vi "Test Harvard pump control.vi"() -> ()   [LabVIEW 2014]
uses:
  <vilib>/Instr/_visa.llb/VISA Configure Serial Port (Instr).vi
panel:
  out "length":i32
  out "error out":errorcluster
  out "read buffer":string
  in  "Send string":string
  in  "stop":bool
  in  "Send string":bool
  out "command string sent":string
  in  "VISA resource name":refnum<visa-resource-name>="COM4"
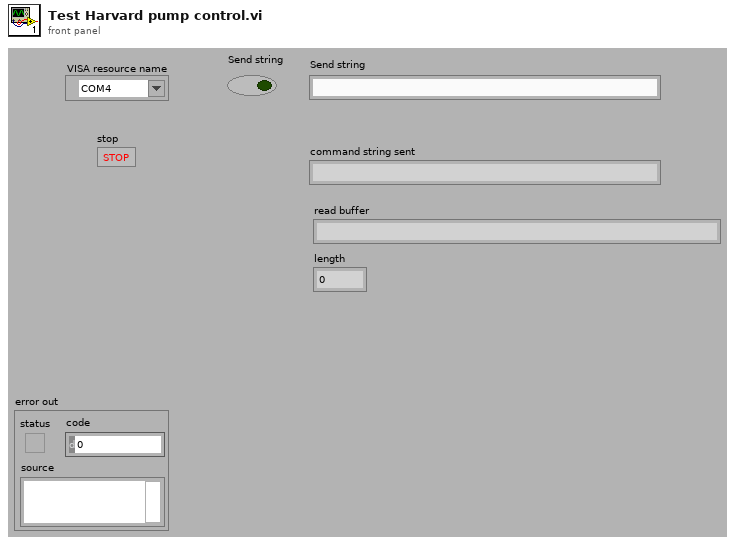
[diagram p1: front panel]
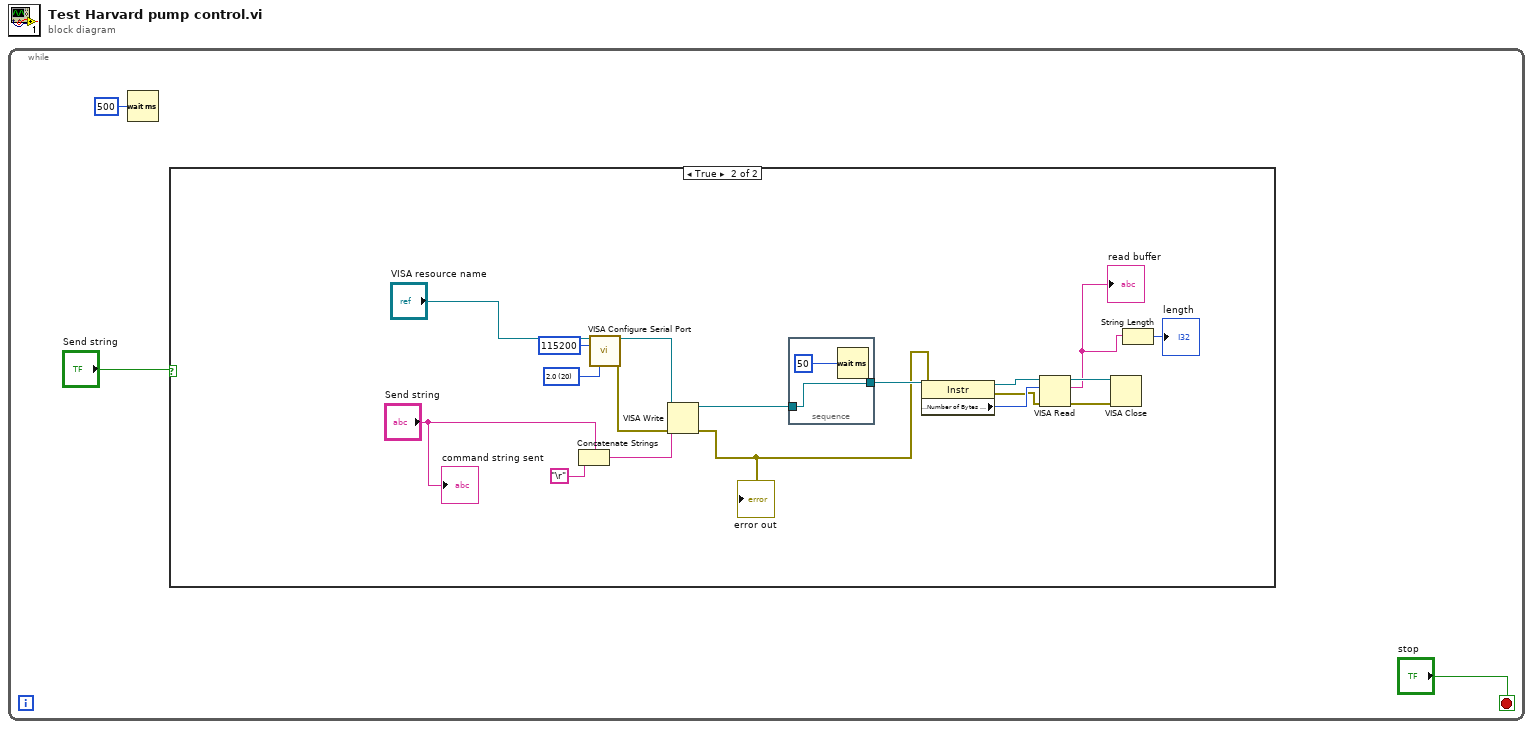
[diagram p0: block diagram]
diagram:
  n1 = while {
    stop <- "stop" stop-if-true
    n2 = Wait (ms)(milliseconds to wait=u32 500) -> ()  [unwired: 1 out]
    n3 = case shown="True" "Send string" {
      frame False {
      }
      frame True {
        w6 = u16 20 items=["1.0"=10, "1.5"=15, "2.0"=20] ("stop bits (10: 1 bit)")
        n4 = Concatenate Strings("Send string", "\r") -> (w16:string)
        n5 = call-poly "VISA Configure Serial Port"("VISA resource name"="VISA resource name", "baud rate (9600)"=u32 115200, "stop bits (10: 1 bit)"=w6) -> ("VISA resource name out"=w15:refnum<visa-resource-name>, "error out"=w14:errorcluster)  [unwired: 4 in, 7 out]
        n6 = VISA Write(VISA resource name=w15, write buffer=w16, error in (no error)=w14) -> (VISA resource name out=w11:refnum<visa-resource-name>, error out=w10:errorcluster)  [unwired: 1 out]
        "error out" <- w10
        n7 = stacked-sequence {
          tunnel: [w22] -> w21
          tunnel: w11 -> [w22]
          frame #0 {
            n8 = Wait (ms)(milliseconds to wait=50) -> ()  [unwired: 1 out]
          }
        }
        n9 = property class="Instr"(reference=w21, error in=w10) -> (reference out=w20:refnum<visa-resource-name>, error out=w18:errorcluster, "Serial Settings:Number of Bytes at Serial Port"=w19:u32)
        n10 = VISA Read(VISA resource name=w20, byte count=w19, error in (no error)=w18) -> (VISA resource name out=w8:refnum<visa-resource-name>, read buffer=w5:string, error out=w9:errorcluster)  [unwired: 1 out]
        "read buffer" <- w5
        n11 = VISA Close(VISA resource name=w8, error in (no error)=w9) -> ()  [unwired: 1 out]
        n12 = String Length(string=w5) -> (length=→"length":i32)
        "command string sent" <- "Send string"
      }
    }
  }
